vi "Sub_Stiffen_Fixed_Beam_Location.vi"(11 "Pre-BC Matrix":dbl[][](array[numeric])) -> (3 "Post-BC Matrix":dbl[][](array[numeric]))   [LabVIEW 2019]
uses:
  <vilib>/Analysis/Matrix/Numeric/Conversions/Matrix To Array - RM.vi
  <vilib>/Analysis/Matrix/NI_Matrix.lvlib
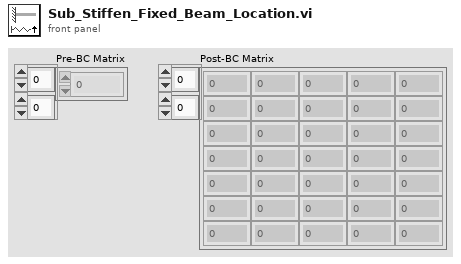
[diagram p1: front panel]
types:
  T1 = typedef "NI_Matrix.lvlib/RealMatrix.ctl" = dbl[][]
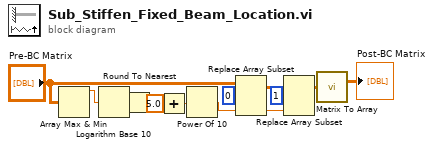
[diagram p0: block diagram]
diagram:
  w10 = 1
  w11 = 0
  n1 = Array Max & Min(array="Pre-BC Matrix") -> (max value=w2:dbl)  [unwired: 3 out]
  n2 = Logarithm Base 10(1:w2) -> (0:w7:dbl)
  n3 = Round To Nearest(number=w7) -> (nearest integer value=w6:dbl)
  n4 = Add(x=w6, y=5.0) -> (x+y=w4:dbl)
  n5 = Power Of 10(x=w4) -> (10^x=w3:dbl)
  n6 = Replace Array Subset(array="Pre-BC Matrix", new element=w3, index (row)=w11, index (col)=w11) -> (w12:T1)
  n7 = Replace Array Subset(array=w12, new element=w3, index (row)=w10, index (col)=w10) -> (w9:T1)
  n8 = call-poly <vilib>:"Matrix To Array.vi"("Real Matrix"=w9) -> ("Real 2D Array"=→"Post-BC Matrix":dbl[][])
